vi "Set Scaling Parameters (Linear).vi"(0 "session in":refnum<k21>, 1 "serial number":string, 2 "password":string, 5 "physical channel":refnum<k21>="$DefaultPhysChans", 7 "slope":dbl, 9 "intercept":dbl, 11 "error in (no error)":errorcluster) -> (4 "session out":refnum<k21>, 6 "physical channel out":refnum<k21>, 15 "error out":errorcluster)   [LabVIEW 2020, in "SLSC.lvlib"]
doc: "Sets scaling parameters for a linear scale that uses the equation y = mx + b, where x is a pre-scaled value and y is a scaled value."
uses:
  <vilib>/SLSC/SLSC.lvlib
  nislsclvapi.dll
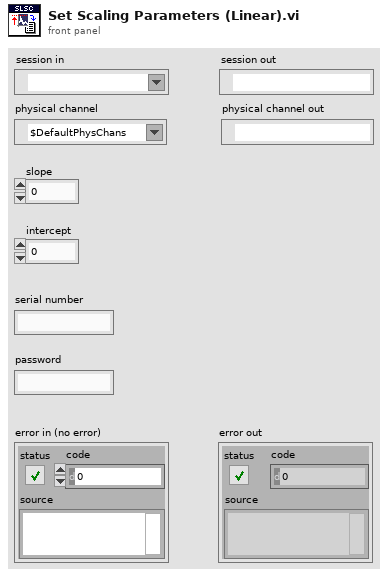
[diagram p1: front panel]
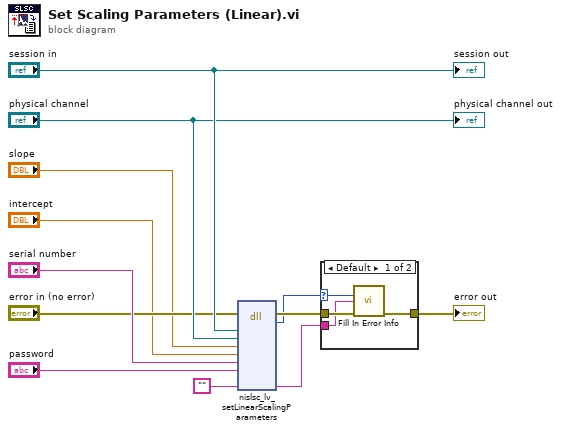
[diagram p0: block diagram]
diagram:
  n1 = dll-call lib="nislsclvapi.*" fn="nislsc_lv_setLinearScalingParameters"(error in="error in (no error)", "session"="session in", "physical channel"="physical channel", "slope"="slope", "intercept"="intercept", "serialNum"="serial number", "password"="password", "extendedErrorInfo"="") -> (error out=w5:errorcluster, "return type"=w4:i32, "extendedErrorInfo"=w2:string)  [unwired: 10 in, 1 out]
  n2 = case shown="Default" w4 {
    selector: w4 -> [w13 _]
    tunnel: w2 -> [w14 _]
    tunnel: w5 -> [w16 w17]
    tunnel: [w15 w17] -> w3
    frame Default {
      n3 = call <vilib>:"Fill In Error Info.vi"("status code"=w13, "extended error info"=w14, "error in"=w16) -> ("error out"=w15:errorcluster)  [unwired: 12 in]
    }
    frame 0 {
    }
  }
  "error out" <- w3
  "session out" <- "session in"
  "physical channel out" <- "physical channel"
